vi "20TVTI-Set-T.vi"(8 "error in (no error)":errorcluster, 10 "20TVTI Control":T1, 11 "Mercury Reference In":T2) -> (0 "error out":errorcluster)   [LabVIEW 2019]
uses:
  Equipment/Mercury iXX/Public/Controls/Mercury Reference.ctl
  Equipment/Mercury iXX/Public/Controls/Comms Transport Layer.ctl
  Equipment/Mercury iXX/Private/Controls/Query Dynamic Reference.ctl
  Gustav/20TVTI_Control.ctl
  Equipment/Mercury iXX/Public/Libraries/System/Open/Open Device.vi
  Equipment/Mercury iXX/Mercury iXX.lvlib
  Equipment/Mercury iXX/Public/Libraries/System.lvlib
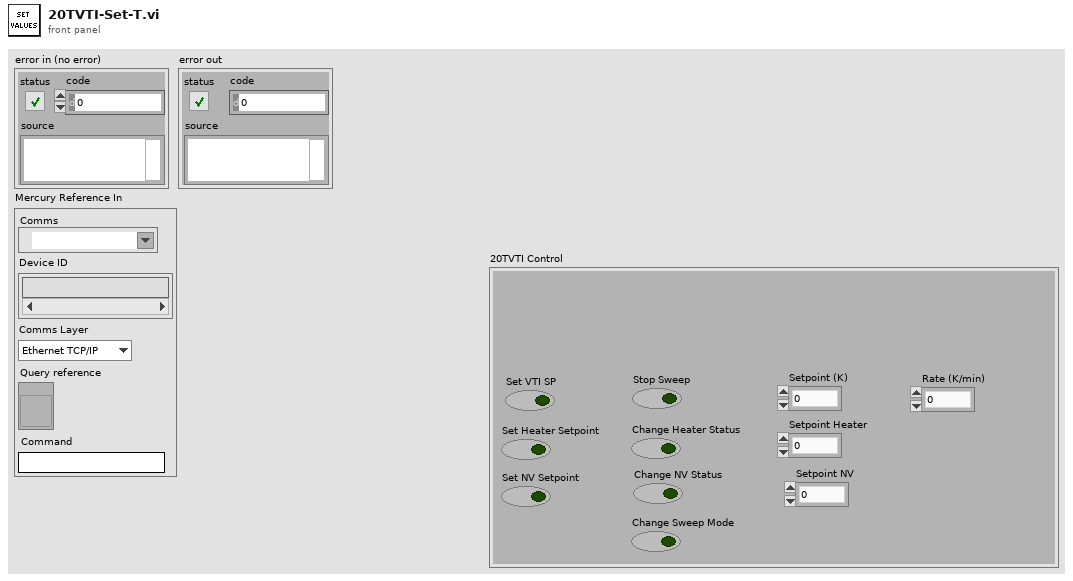
[diagram p1: front panel]
types:
  T1 = typedef "20TVTI_Control.ctl" = cluster{"Set VTI SP":bool, "Change NV Status":bool, "Set NV Setpoint":bool, "Change Heater Status":bool, "Set Heater Setpoint":bool, "Stop Sweep":bool, "Setpoint (K)":dbl, "Rate (K/min)":dbl, "Setpoint Heater":dbl, "Setpoint NV":dbl, "Change Sweep Mode":bool}
  T2 = typedef "Mercury iXX.lvlib/Mercury Reference.ctl" = cluster{"Comms":refnum<visa-resource-name>, "Device ID":string[], "Comms Layer":T3, "Command":string, "Query reference":T4}
  T3 = typedef "Mercury iXX.lvlib/Comms Transport Layer.ctl" = enum16{"Ethernet TCP/IP", "USB", "ISOBus - RS-232", "GPIB"}
  T4 = typedef "Mercury iXX.lvlib/Query Dynamic Reference.ctl" = refnum<vi>
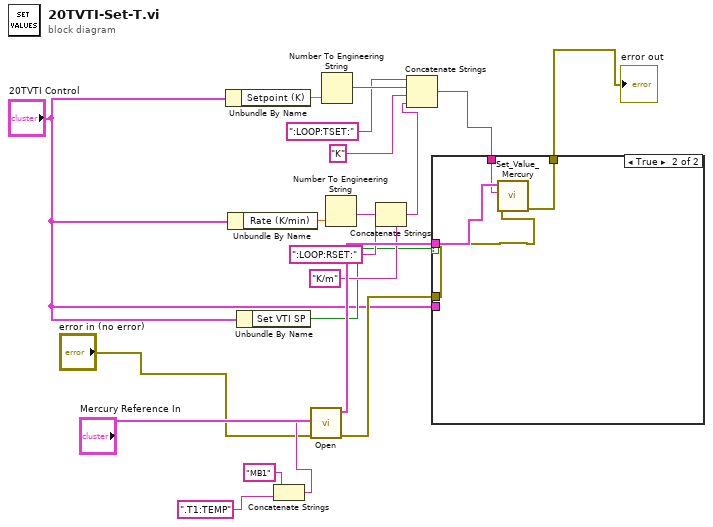
[diagram p0: block diagram]
diagram:
  n1 = Unbundle By Name("20TVTI Control") -> ("Setpoint (K)"=w16:dbl)
  n2 = Unbundle By Name("20TVTI Control") -> ("Rate (K/min)"=w12:dbl)
  n3 = Unbundle By Name("20TVTI Control") -> ("Set VTI SP"=w9:bool)
  n4 = Concatenate Strings("MB1", ".T1:TEMP" ("Device Identifier")) -> (w7:string)
  n5 = call-poly "Open.vi"("error in (no error)"="error in (no error)", "Device Identifier"=w7, "Mercury Reference In"="Mercury Reference In") -> ("error out"=w18:errorcluster, "Mercury Reference Out"=w19:T2)  [unwired: 2 in, 5 out]
  n6 = Number To Engineering String(4:w16) -> (0:w17:string)  [unwired: 3 in]
  n7 = Number To Engineering String(4:w12) -> (0:w13:string)  [unwired: 3 in]
  n8 = Concatenate Strings(":LOOP:RSET:", w13, "K/m") -> (w5:string)
  n9 = Concatenate Strings(":LOOP:TSET:", w17, "K", w5) -> (w6:string)
  n10 = case shown="True" w9 {
    tunnel: w19 -> [_ w25]
    tunnel: w18 -> [w21 w22]
    tunnel: [w21 w23] -> w3
    tunnel: w6 -> [_ w24]
    tunnel: "20TVTI Control" -> [_ _]
    frame False {
    }
    frame True {
      n11 = call "Set_Value_Mercury.vi"("error in"=w22, "Noun(s)"=w24, "Mercury Reference In"=w25) -> ("error out"=w23:errorcluster)  [unwired: 7 in, 1 out]
    }
  }
  "error out" <- w3
